vi "Set Address.vi"(8 "error in (no error)":errorcluster, 10 "Address":string, 11 "File Transfer Behavior in":refnum<class "File Transfer Behavior.lvclass">) -> (0 "error out":errorcluster, 3 "File Transfer Behavior out":refnum<class "File Transfer Behavior.lvclass">)   [LabVIEW 2015, in "RT Management.lvlib" / "File Transfer Behavior.lvclass"]
uses:
  File Transfer Behavior.lvclass
  File Transfer Behavior.lvclass/File Transfer Behavior.ctl
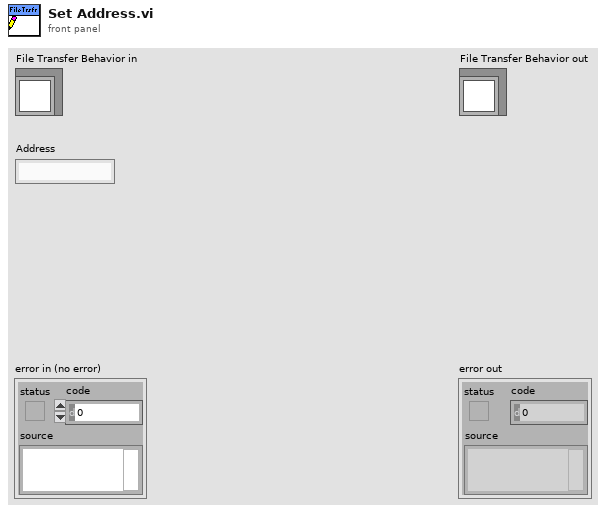
[diagram p1: front panel]
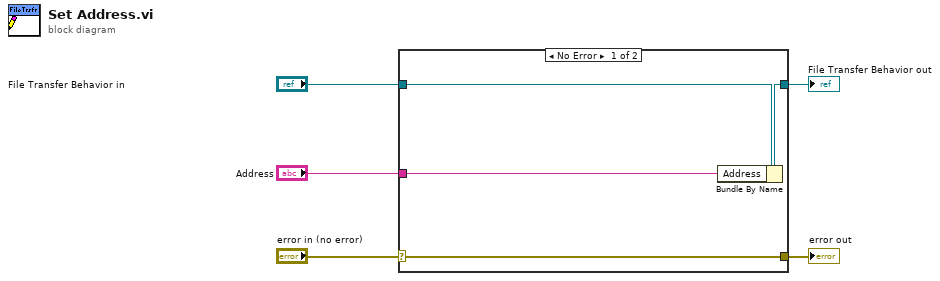
[diagram p0: block diagram]
diagram:
  n1 = case shown="No Error" "error in (no error)" {
    selector: "error in (no error)" -> [w9 w10]
    tunnel: [w9 w10] -> w4
    tunnel: [w7 w11] -> w2
    tunnel: "File Transfer Behavior in" -> [w8 w11]
    tunnel: "Address" -> [w6 _]
    frame No Error {
      n2 = Bundle By Name(cluster=w8, "Address"=w6) -> (w7:refnum<class "File Transfer Behavior.lvclass">)
    }
    frame Error {
    }
  }
  "error out" <- w4
  "File Transfer Behavior out" <- w2
